vi "CmdExe.Ping Host.vi"(10 "Timeout":i32=200, 11 "Host":string) -> (3 "Found":bool)   [LabVIEW 2019]
panel:
  out "return code":i32
  out "standard error":string
  out "standard output":string
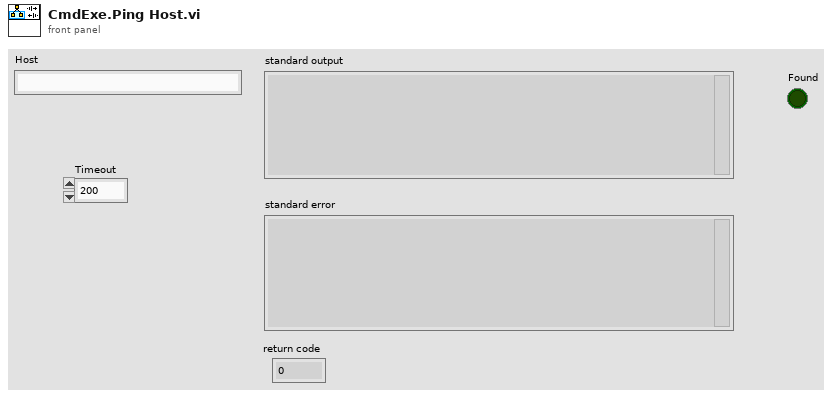
[diagram p1: front panel]
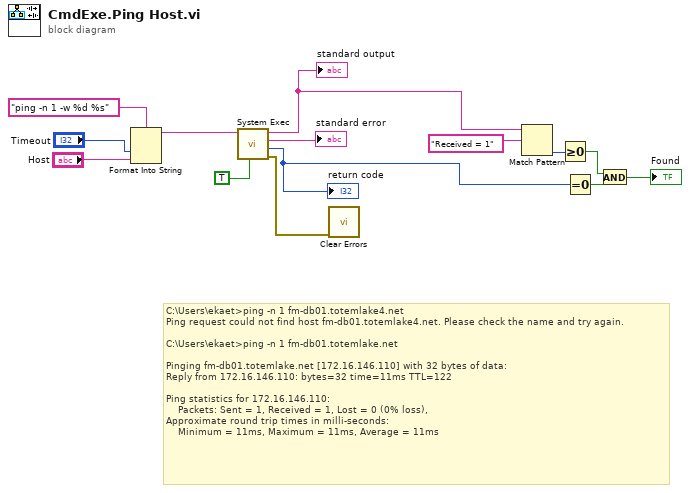
[diagram p0: block diagram]
diagram:
  # "C:\\Users\\ekaet>ping -n 1 fm-db01.totemlake4.net\nPing request could not find host fm-db01.totemlake4.net. Please check the name and try again.\n\nC:\\Users\\ekaet>ping -n 1 fm-db01.totemlake.net\n\nPinging fm-db01.totemlake.net [172.16.146.110] with 32 bytes of data:\nReply from 172.16.146.110: bytes=32 time=11ms TTL=122\n\nPing statistics for 172.16.146.110:\n    Packets: Sent = 1, Received = 1, Lost = 0 (0% loss),\nApproximate round trip times in milli-seconds:\n    Minimum = 11ms, Maximum = 11ms, Average = 11ms"
  n1 = Format Into String(format string="ping -n 1 -w %d %s", "Timeout", "Host") -> (resulting string=w12:string)  [unwired: 2 in, 1 out]
  n2 = call <vilib>:"System Exec.vi"("run minimized? (F)"=TRUE, "command line"=w12) -> ("error out"=w10:errorcluster, "return code"=w2:i32, "standard error"=→"standard error":string, "standard output"=w9:string)  [unwired: 6 in]
  "standard output" <- w9
  "return code" <- w2
  n3 = call <vilib>:"Clear Errors.vi"("error in (no error)"=w10) -> ()  [unwired: 5 in, 2 out]
  n4 = Match Pattern(string=w9, regular expression="Received = 1") -> (offset past match=w7:i32)  [unwired: 1 in, 3 out]
  n5 = Greater Or Equal To 0?(x=w7) -> (x >= 0?=w4:bool)
  n6 = Equal To 0?(x=w2) -> (x = 0?=w3:bool)
  n7 = And(x=w4, y=w3) -> (x .and. y?=→"Found":bool)
